vi "GrabFrame.vi"(4 "IMAQ Session Out":refnum<k11>, 5 "error in":errorcluster, 6 "Stop":bool caption="Stop (F)", 7 "Saving":bool=TRUE, 8 "New Image":T1) -> (0 "error out":errorcluster, 1 "Stopped":bool, 2 "Image Pixels (U16)":u16[][](array[numeric]))   [LabVIEW 2017]
doc: "Creates, and edits acquisitions using the NI Vision Acquisition Express VI.\n\nThe NI Vision Acquisition Wizard is launched by placing the Express VI on the block diagram. Select an acquisition source and configure an acquisition using NI-IMAQ, NI-IMAQdx, or simulate an acquisition by reading an AVI or image files from a folder. After an acquisition is configured, select controls and indicators to be able to programmatically set in LabVIEW. Double-click the Vision Acquisition Express VI to edit the acquisition.\n\nNote: Any images created by the Express VI need to be disposed after use. Use the IMAQ Dispose.vi to cleanup the images output by the Express VI when they are no longer needed."
uses:
  <vilib>/vision/Image Controls.llb/IMAQ Image.ctl
  <vilib>/Utility/file.llb/Write Delimited Spreadsheet (I64).vi
  <resource>/objmgr/IMAQImage.rc
panel:
  out "Processed Frames/s":dbl
  out "Acquired FPS":dbl format="%#_3g"
  out "debugging error":errorcluster
  out "Acquired Buffer Number":u32
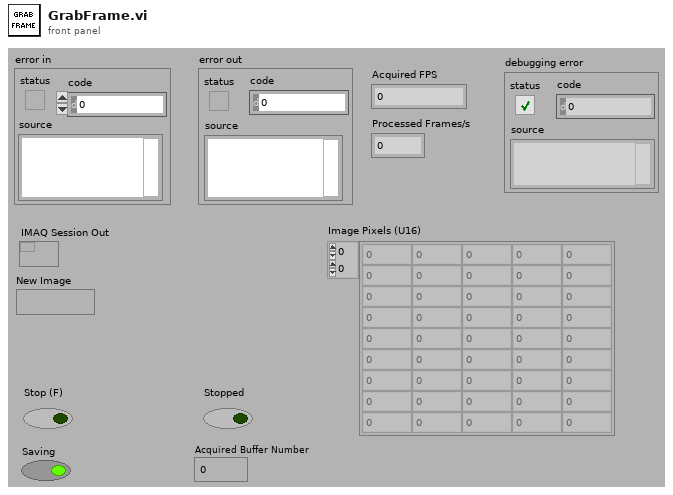
[diagram p1: front panel]
types:
  T1 = typedef "IMAQ Image.ctl" = refnum<image>
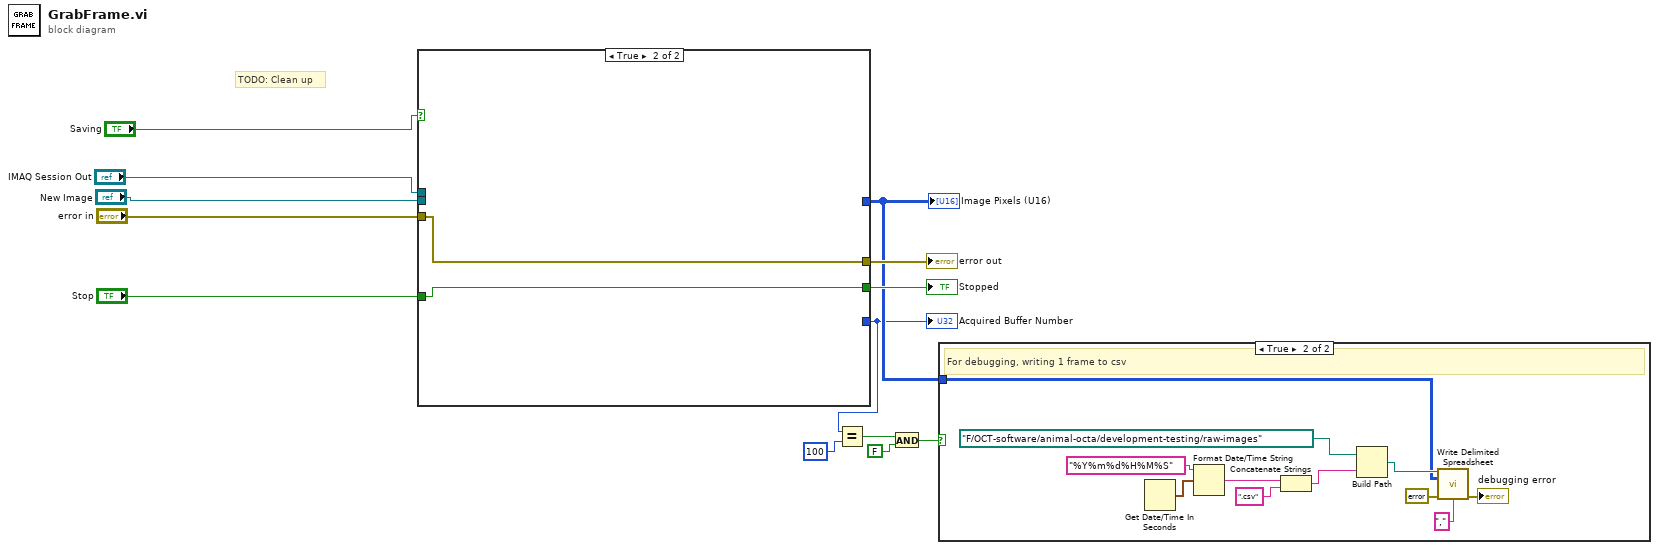
[diagram p0: block diagram]
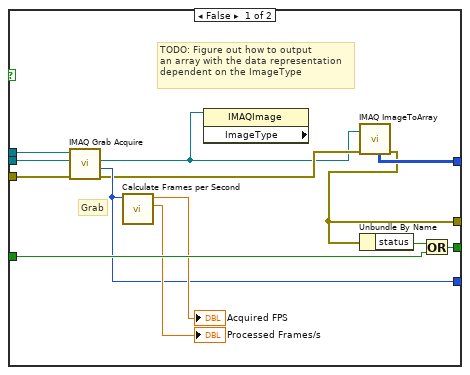
[diagram p2: hidden frame]
diagram:
  # "TODO: Clean up"
  n1 = case shown="True" "Saving" {
    tunnel: "Stop" -> [w25 w28]
    tunnel: "IMAQ Session Out" -> [w24 _]
    tunnel: "New Image" -> [w23 _]
    tunnel: [w15 w27] -> w12
    tunnel: [w20 w28] -> w7
    tunnel: [w19 _] -> w6
    tunnel: [w18 _] -> w5
    tunnel: "error in" -> [w17 w27]
    frame False {
      # "TODO: Figure out how to output\nan array with the data representation\ndependent on the ImageType"
      # "Grab"
      n2 = call <vilib>:"IMAQ Grab Acquire.vi"("error in (no error)"=w17, "Image In"=w23, "IMAQ Session In"=w24) -> ("error out"=w16:errorcluster, "Acquired Buffer Number"=w18:u32, "Image Out"=w14:T1)  [unwired: 1 in, 5 out]
      n3 = call <vilib>:"Calculate Frames per Second.vi"("Buffer Number"=w18) -> ("Processed Frames/s"=→"Processed Frames/s":dbl, "Acquired Frames/s"=→"Acquired FPS":dbl)  [unwired: 8 in, 1 out]
      n4 = property class="IMAQImage" props=["ImageType"](reference=w14) -> ()  [unwired: 1 in, 3 out]
      n5 = call "IMAQ ImageToArray"("error in (no error)"=w16, "Image"=w14) -> ("Image Pixels (U16)"=w19:u16[][], "error out"=w15:errorcluster)  [unwired: 2 in, 3 out]
      n6 = Unbundle By Name(w15) -> ("status"=w26:bool)
      n7 = Or(x=w26, y=w25) -> (x .or. y?=w20:bool)
    }
    frame True {
    }
  }
  "Stopped" <- w7
  "error out" <- w12
  "Acquired Buffer Number" <- w5
  "Image Pixels (U16)" <- w6
  n8 = Equal?(x=w5, y=u32 100) -> (x = y?=w9:bool)
  n9 = And(x=w9, y=FALSE) -> (x .and. y?=w8:bool)
  n10 = case shown="True" w8 {
    tunnel: w6 -> [_ w32]
    frame False {
    }
    frame True {
      # "For debugging, writing 1 frame to csv"
      n11 = Get Date/Time In Seconds() -> (seconds since 1Jan1904=w36:timestamp)
      n12 = Format Date/Time String(time format string (%c)="%Y%m%d%H%M%S", seconds (now)=w36) -> (date/time string=w37:string)  [unwired: 1 in]
      n13 = Concatenate Strings(w37, ".csv" ("string")) -> (w38:string)
      n14 = Build Path(base path=path "F:/OCT-software/animal-octa/development-testing/raw-images", name or relative path=w38) -> (appended path=w39:path)
      n15 = call-poly <vilib>:"Write Delimited Spreadsheet.vi"("file path (dialog if empty)"=w39, "2D data"=w32, "error in (no error)"=errorcluster {"status"=FALSE, "code"=0, "source"=""}, "delimiter (\\t)"="," ("delimiter (\\t)")) -> ("error out"=→"debugging error":errorcluster)  [unwired: 10 in, 1 out]
    }
  }
